vi "QI_proto.vi"(4 "Y_base":sgl, 5 "sample(quar)":i32=12, 6 "X_base":sgl, 7 "R_step":dbl=0.4, 8 "修正次数":i32=1, 10 "Centroid":cluster{"X Centroid":sgl, "Y Centroid":sgl} {"Y Centroid" format="%.2f"; "X Centroid" format="%.2f"}, 11 "ROI array":dbl[][](array[numeric])) -> (1 "array R":dbl[](array[numeric]), 2 "xc and yc":cluster{"X Centroid":sgl, "Y Centroid":sgl} {"Y Centroid" format="%.2f"; "X Centroid" format="%.2f"}, 3 "radial profile array":dbl[](array[numeric]))   [LabVIEW 2017]
doc: "使用该模板构建标准状态机设计模式。各状态执行代码并决定转移状态。将该设计模式与根据用户动作响应而执行代码的用户界面事件处理器模式相比较。同时将该设计模式与每段消息处理代码可以将零至多个新消息加入队列的队列消息处理器模式相比较。\n注：该模板的设计未遵守最新NI推荐的编程风格。请通过“创建项目”对话框（而不要采用该模板），创建基于项目的标准状态机模式的完整实现。"
uses:
  QI state.ctl
panel:
  out "dy1":dbl
  out "dx1":dbl
  out "dy2":dbl
  out "dx2":dbl
  out "radial profile":dbl[][](graph)
  in  "QI 传递变量":T1
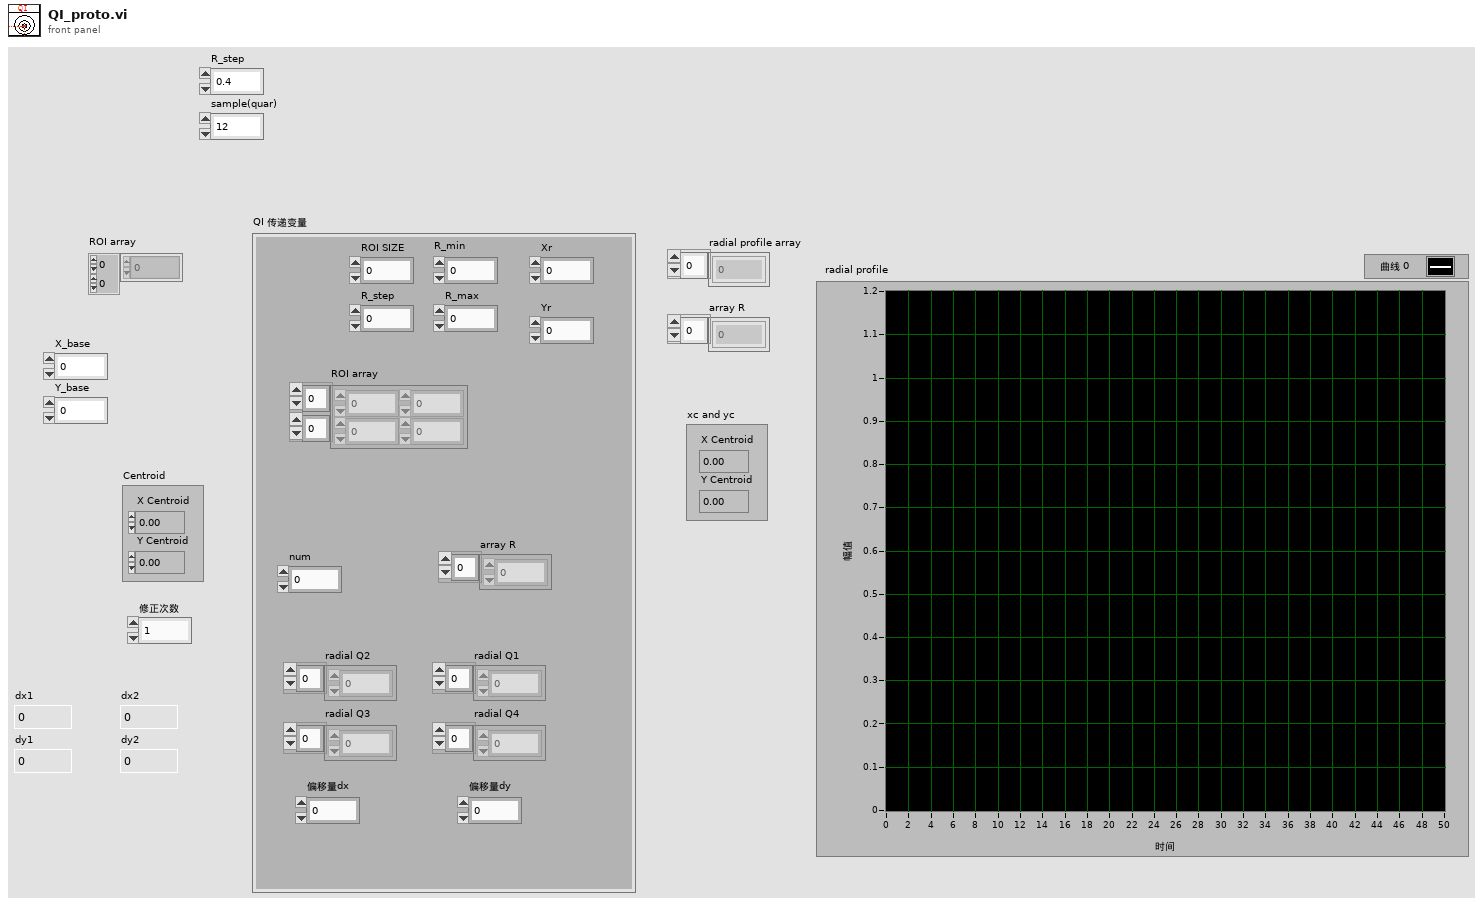
[diagram p1: front panel]
types:
  T1 = typedef "QI 传递变量.ctl" = cluster{"ROI SIZE":i32, "R_step":dbl, "R_min":dbl, "R_max":dbl, "num":dbl, "array R":dbl[], "radial Q1":dbl[], "radial Q2":dbl[], "radial Q3":dbl[], "radial Q4":dbl[], "偏移量dx":dbl, "偏移量dy":dbl, "ROI array":sgl[][], "Xr":dbl, "Yr":dbl}
  T2 = typedef "QI state.ctl" = enum16{"初始化", "径向分布", "相关性分析XY", "修正XY", "输出", "错误处理"}
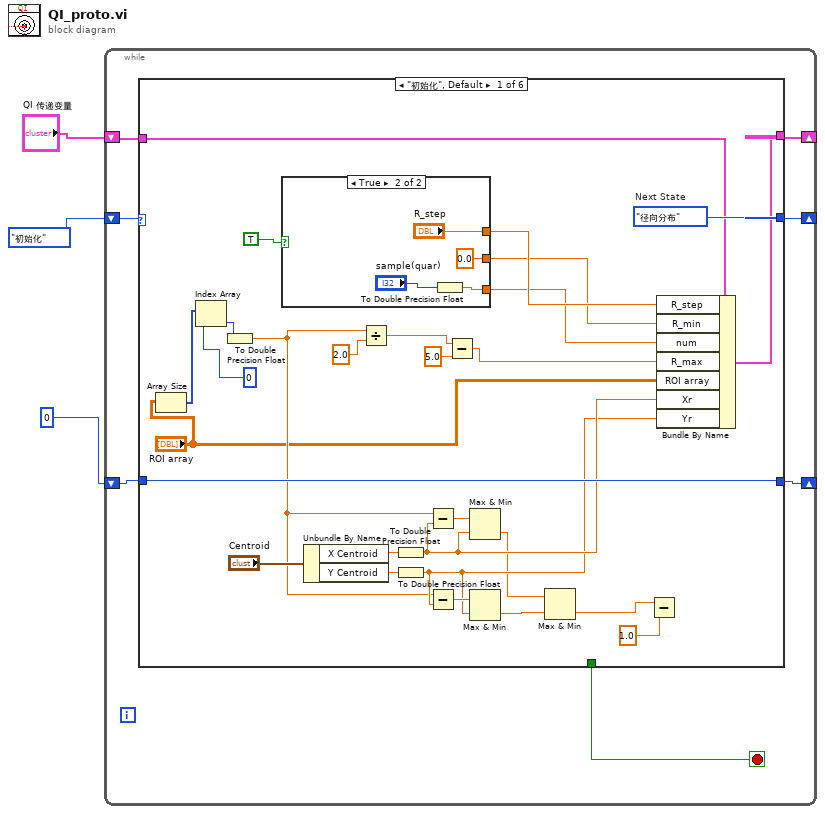
[diagram p0: block diagram]
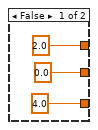
[diagram p2: hidden frame]
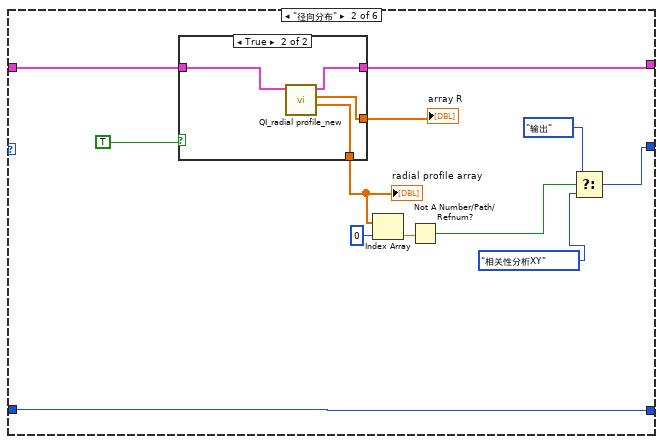
[diagram p3: hidden frame]
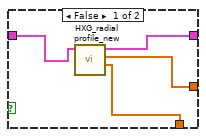
[diagram p4: hidden frame]
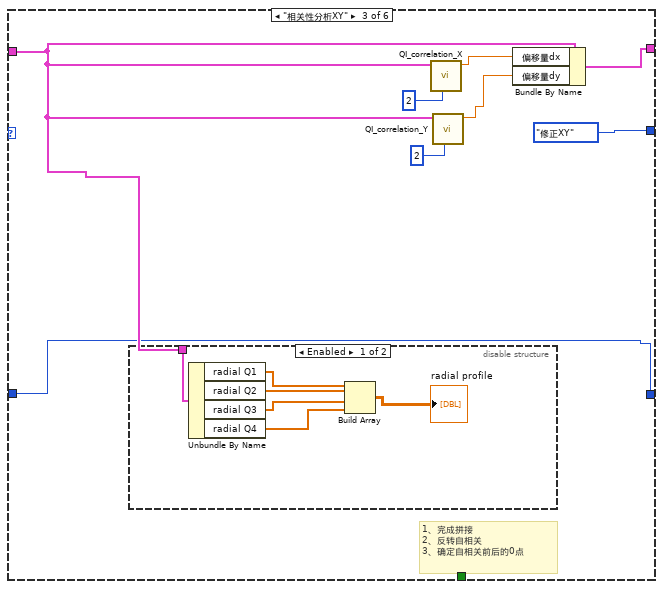
[diagram p5: hidden frame]
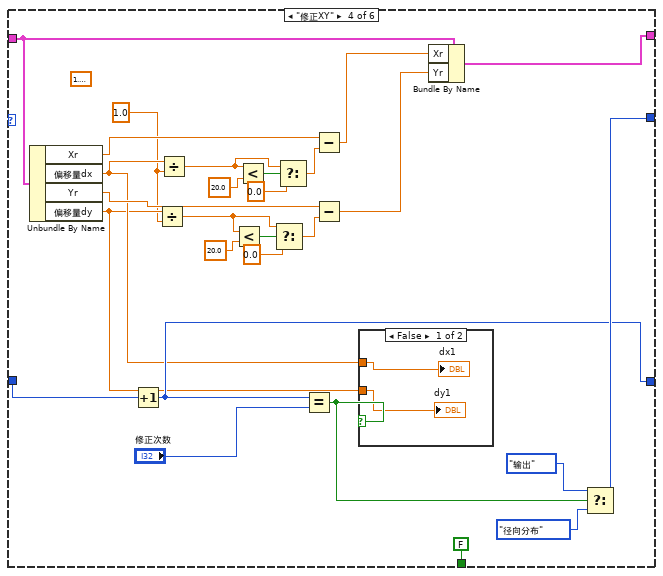
[diagram p7: hidden frame]
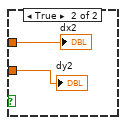
[diagram p8: hidden frame]
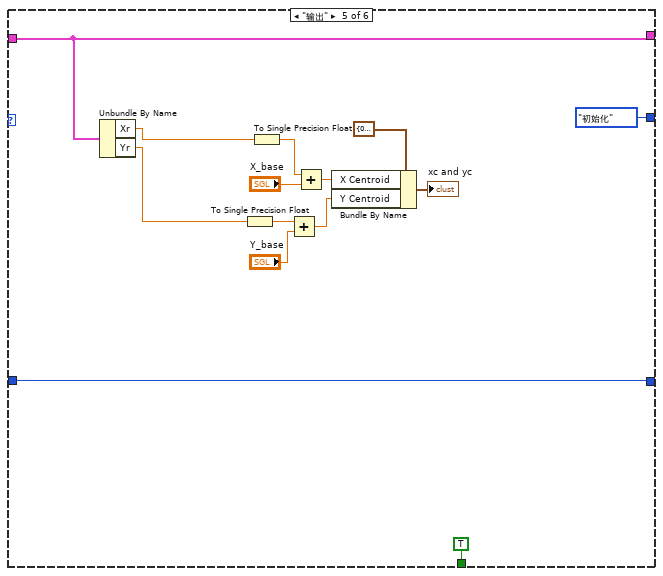
[diagram p9: hidden frame]
diagram:
  n1 = while {
    shift-right: [w9] -> _
    shift-left: QI_state."初始化" ("Beginning State") -> [w10]
    shift-right: [w7] -> _
    shift-left: "QI 传递变量" -> [w8]
    shift-right: [w5] -> _
    shift-left: 0 -> [w6]
    stop <- w4 stop-if-true
    n2 = case shown="\"初始化\", Default" w10 {
      tunnel: [w38 w47 QI_state."修正XY" ("Next State") w103 QI_state."初始化" ("Next State") _] -> w9
      tunnel: w8 -> [w37 w53 w67 w98 w115 w126]
      tunnel: [w36 w57 w72 w97 w115 w126] -> w7
      tunnel: w6 -> [w29 w55 w66 w100 w124 w125]
      tunnel: [w29 w55 w66 w99 w124 w125] -> w5
      tunnel: [_ _ _ FALSE TRUE _] -> w4
      frame "初始化", Default {
        w38 = QI_state."径向分布"  # Next State
        n3 = Array Size(array="ROI array") -> (size(s)=w26:i32[])
        n4 = Index Array(array=w26, index=0 ("索引")) -> (element=w24:i32)
        n5 = To Double Precision Float(number=w24) -> (double precision float=w15:dbl)
        n6 = case shown="True" TRUE {
          tunnel: [2.0 ("R_step") "R_step"] -> w35
          tunnel: [0.0 ("R_min") 0.0 ("R_min")] -> w34
          tunnel: [4.0 ("num") w42] -> w28
          frame False {
          }
          frame True {
            n7 = To Double Precision Float(number="sample(quar)") -> (double precision float=w42:dbl)
          }
        }
        n8 = Unbundle By Name("Centroid") -> ("X Centroid"=w31:sgl, "Y Centroid"=w30:sgl)
        n9 = Divide(x=w15, y=2.0) -> (x/y=w13:dbl)
        n10 = To Double Precision Float(number=w31) -> (double precision float=w22:dbl)
        n11 = To Double Precision Float(number=w30) -> (double precision float=w20:dbl)
        n12 = Subtract(x=w15, y=w22) -> (x-y=w23:dbl)
        n13 = Subtract(x=w15, y=w20) -> (x-y=w21:dbl)
        n14 = Subtract(x=w13, y=5.0) -> (x-y=w12:dbl)
        n15 = Max & Min(x=w23, y=w22) -> (min(x,y)=w19:dbl)  [unwired: 1 out]
        n16 = Max & Min(x=w21, y=w20) -> (min(x,y)=w18:dbl)  [unwired: 1 out]
        n17 = Max & Min(x=w19, y=w18) -> (min(x,y)=w17:dbl)  [unwired: 1 out]
        n18 = Subtract(x=w17, y=1.0) -> ()  [unwired: 1 out]
        n19 = Bundle By Name(cluster=w37, "R_step"=w35, "R_min"=w34, "num"=w28, "R_max"=w12, "ROI array"="ROI array", "Xr"=w22, "Yr"=w20) -> (w36:T1)
      }
      frame "径向分布" {
        n20 = case shown="True" TRUE {
          tunnel: [w60 w64] -> w57
          tunnel: w53 -> [w61 w65]
          tunnel: [w59 w63] -> w56
          tunnel: [w58 w62] -> w52
          frame False {
            n21 = call "HXG_radial profile_new.vi"("QI 传递变量输入"=w61) -> ("radial profile"=w58:dbl[], "array R"=w59:dbl[], "QI 传递变量输出"=w60:T1)  [unwired: 8 in]
          }
          frame True {
            n22 = call "QI_radial profile_new.vi"("QI 传递变量输入"=w65) -> ("radial profile"=w62:dbl[], "array R"=w63:dbl[], "QI 传递变量输出"=w64:T1)  [unwired: 8 in]
          }
        }
        "radial profile array" <- w52
        "array R" <- w56
        n23 = Index Array(array=w52, index=0 ("索引")) -> (element=w50:dbl)
        n24 = Not A Number/Path/Refnum?(number/path/refnum=w50) -> (NaN/Path/Refnum?=w49:bool)
        n25 = Select(t=QI_state."输出" ("Next State"), s=w49, f=QI_state."相关性分析XY" ("Next State")) -> (s? t:f=w47:T2)
      }
      frame "相关性分析XY" {
        # "1、完成拼接\n2、反转自相关\n3、确定自相关前后的0点"
        n26 = disable-structure shown="Enabled" {
          disable-tunnel: w67 -> [w74 _]
          frame Enabled {
            n27 = Unbundle By Name(w74) -> ("radial Q1"=w79:dbl[], "radial Q2"=w78:dbl[], "radial Q3"=w77:dbl[], "radial Q4"=w76:dbl[])
            n28 = Build Array(w79, w78, w77, w76) -> (→"radial profile":dbl[][])
          }
          frame Disabled {
          }
        }
        n29 = call "QI_correlation_X.vi"("拟合半径"=2, "QI 传递变量"=w67) -> ("最相关位置"=w69:dbl)  [unwired: 9 in]
        n30 = call "QI_correlation_Y.vi"("拟合半径"=2, "QI 传递变量"=w67) -> ("最相关位置"=w71:dbl)  [unwired: 9 in]
        n31 = Bundle By Name(cluster=w67, "偏移量dx"=w69, "偏移量dy"=w71) -> (w72:T1)
      }
      frame "修正XY" {
        w80 = 1.0 ("y")
        (unwired) 1.5707963267948966
        n32 = Unbundle By Name(w98) -> ("Xr"=w105:dbl, "偏移量dx"=w93:dbl, "Yr"=w106:dbl, "偏移量dy"=w92:dbl)
        n33 = Increment(x=w100) -> (x+1=w99:i32)
        n34 = Divide(x=w92, y=w80) -> (x/y=w83:dbl)
        n35 = Divide(x=w93, y=w80) -> (x/y=w89:dbl)
        n36 = Less?(x=w83, y=20.0) -> (x < y?=w85:bool)
        n37 = Less?(x=w89, y=20.0) -> (x < y?=w90:bool)
        n38 = Select(t=w83, s=w85, f=0.0) -> (s? t:f=w82:dbl)
        n39 = Select(t=w89, s=w90, f=0.0) -> (s? t:f=w87:dbl)
        n40 = Equal?(x=w99, y="修正次数") -> (x = y?=w94:bool)
        n41 = Subtract(x=w105, y=w87) -> (x-y=w96:dbl)
        n42 = Subtract(x=w106, y=w82) -> (x-y=w95:dbl)
        n43 = case shown="False" w94 {
          tunnel: w93 -> [w108 w110]
          tunnel: w92 -> [w107 w109]
          frame False {
            "dx1" <- w108
            "dy1" <- w107
          }
          frame True {
            "dx2" <- w110
            "dy2" <- w109
          }
        }
        n44 = Bundle By Name(cluster=w98, "Xr"=w96, "Yr"=w95) -> (w97:T1)
        n45 = Select(t=QI_state."输出", s=w94, f=QI_state."径向分布" ("Next State")) -> (s? t:f=w103:T2)
      }
      frame "输出" {
        n46 = Unbundle By Name(w115) -> ("Xr"=w114:dbl, "Yr"=w113:dbl)
        n47 = To Single Precision Float(number=w113) -> (single precision float=w118:sgl)
        n48 = To Single Precision Float(number=w114) -> (single precision float=w120:sgl)
        n49 = Add(x=w118, y="Y_base") -> (x+y=w119:sgl)
        n50 = Add(x=w120, y="X_base") -> (x+y=w122:sgl)
        n51 = Bundle By Name(cluster=cluster{"X Centroid":sgl, "Y Centroid":sgl} {"X Centroid"=0.0, "Y Centroid"=0.0} ("xc and yc 2"), "X Centroid"=w122, "Y Centroid"=w119) -> (→"xc and yc":cluster{"X Centroid":sgl, "Y Centroid":sgl})
      }
      frame "错误处理" {
      }
    }
  }
